vi "p185.vi"() -> ()   [LabVIEW 2017]
panel:
  out "Waveform Chart":dbl(graph)
  out "error out":errorcluster
  in  "error in (no error)":errorcluster
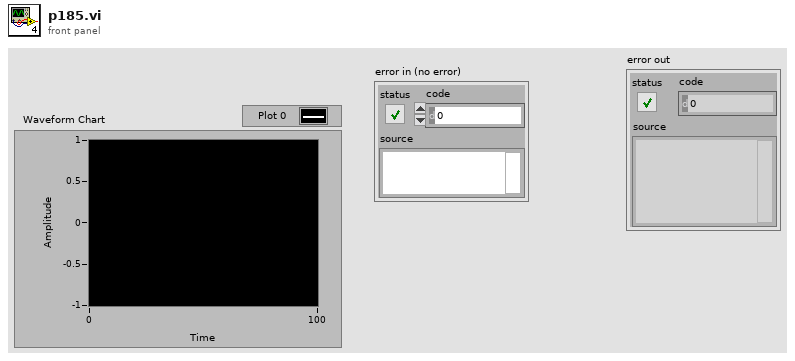
[diagram p1: front panel]
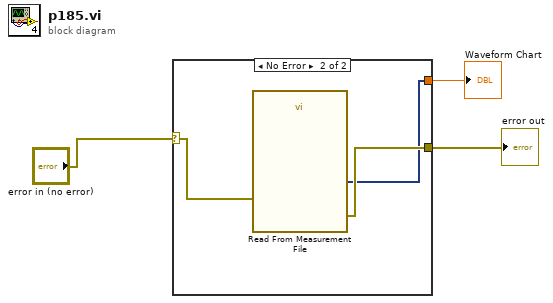
[diagram p0: block diagram]
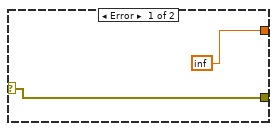
[diagram p2: hidden frame]
diagram:
  n1 = case shown="No Error" "error in (no error)" {
    selector: "error in (no error)" -> [w5 w7]
    tunnel: [w5 w8] -> w2
    tunnel: [inf w6] -> w1
    frame Error {
    }
    frame No Error {
      n2 = call "Read From Measurement File"("error in (no error)"=w7) -> ("error out"=w8:errorcluster, "Signals"=w6:dynamicdata)  [unwired: 5 in, 4 out]
    }
  }
  "error out" <- w2
  "Waveform Chart" <- w1
